vi "Fetch_chirp_waveform_optimized.vi"(0 "VISA resource name":refnum<visa-resource-name>, 11 "error in (no error)":errorcluster) -> (4 "VISA resource name out":refnum<visa-resource-name>, 6 "Waveform Data":waveform(dbl)(graph), 12 "overall meas time":u32, 15 "error out":errorcluster)   [LabVIEW 2011]
doc: "Returns the waveform that an oscilloscope acquires for a channel you specify. An acquisition that you initiate before calling this VI generates the waveform.\n\nYou first enable channels with the Configure Channel VI. Then you use the Initiate VI to start an acquisition on the enabled channels. An oscilloscope concurrently acquires waveforms for these channels. You must call the Fetch Waveform VI separately to obtain waveforms for each enabled channel. However, you also can call the Read Waveform VI instead of using the above low-level VIs.\n\n<B>Note:</B> Use the Fetch Waveform VI only with other low-level VIs, such as the Initiate VI, the Abort VI, and the Fetch Waveform Measurement VI. High-level VIs such as the Read Waveform VI automatically incorporate the functions of the Initiate VI and the Fetch Waveform VI. The Fetch Waveform VI does not check the status of an instrument."
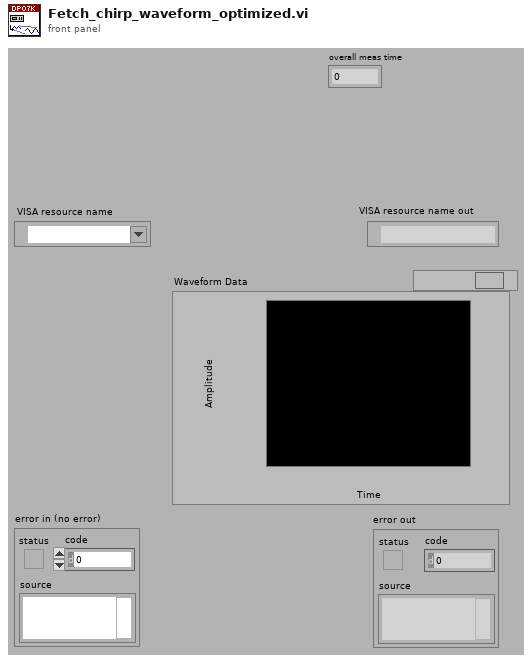
[diagram p1: front panel]
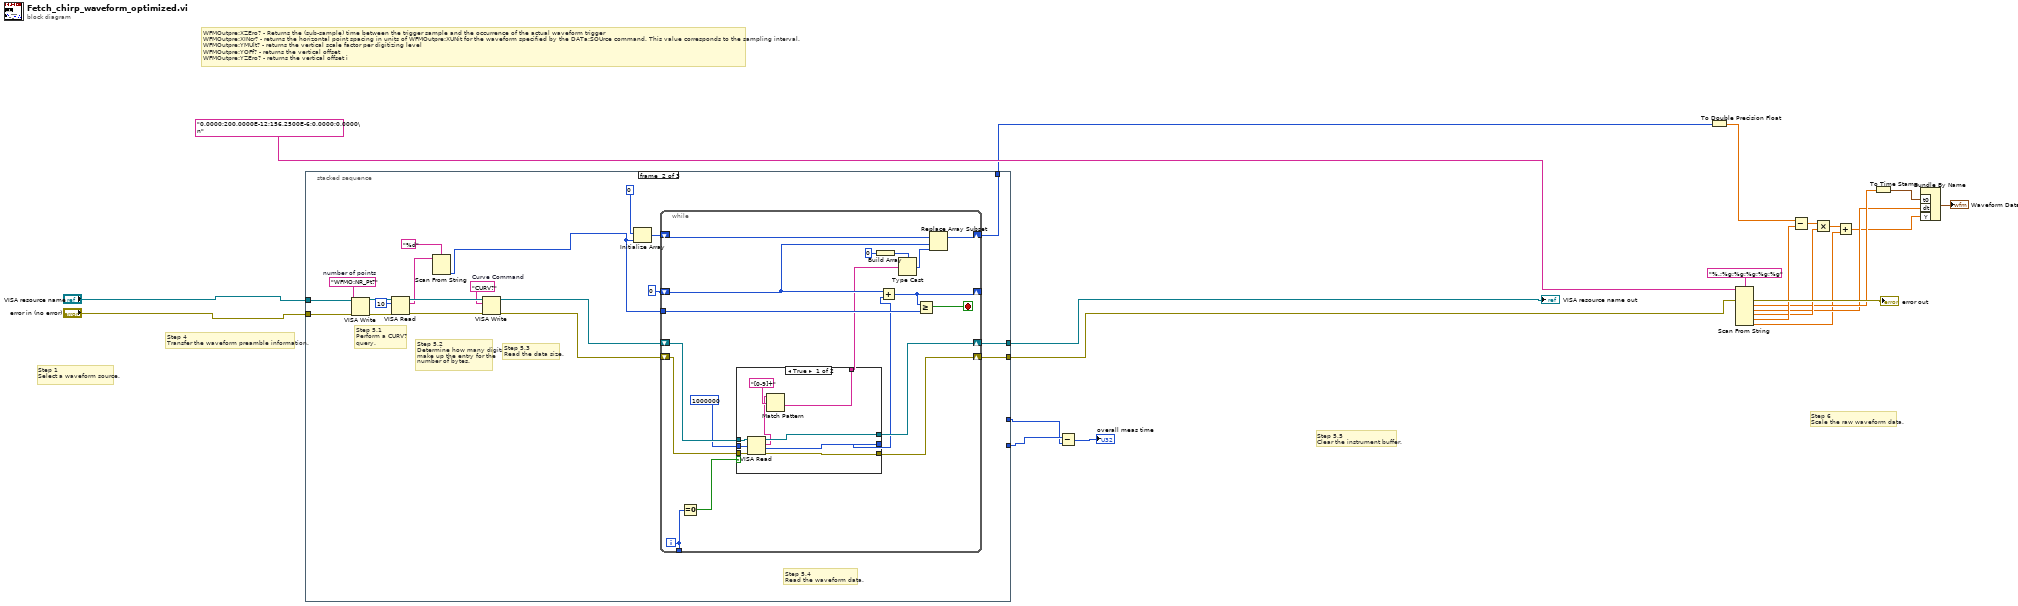
[diagram p0: block diagram]
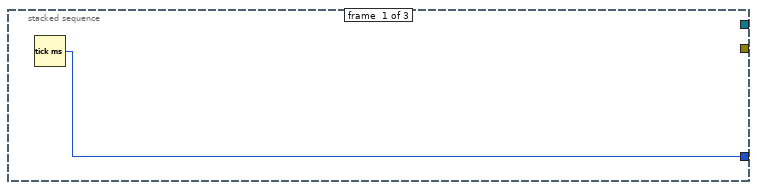
[diagram p2: hidden frame]
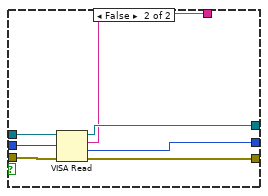
[diagram p3: hidden frame]
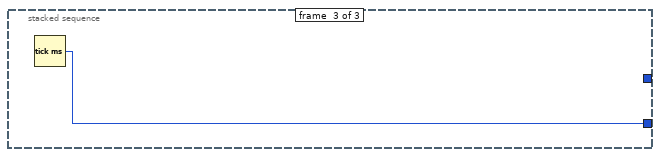
[diagram p4: hidden frame]
diagram:
  # "WFMOutpre:XZEro? - Returns the (sub-sample) time between the trigger sample and the occurrence of the actual waveform trigger\nWFMOutpre:XINcr? - returns the horizontal point spacing in units of WFMOutpre:XUNit for the waveform specified by the DATa:SOUrce command. This value corresponds to the sampling interval.\nWFMOutpre:YMUlt? - returns the vertical scale factor per digitizing level \nWFMOutpre:YOFf? - returns the vertical offset \nWFMOutpre:YZEro? - returns the vertical offset i"
  # "Step 1       \nSelect a waveform source."
  # "Step 6    \nScale the raw waveform data."
  # "Step 5.5    \nClear the instrument buffer."
  # "Step 4\nTransfer the waveform preamble information."
  n1 = stacked-sequence {
    tunnel: [_ w43 _] -> w21
    tunnel: [_ w42 _] -> w20
    tunnel: [_ w38 _] -> w18
    tunnel: "VISA resource name" -> [_ w37 _]
    tunnel: "error in (no error)" -> [_ w36 _]
    tunnel: [w23 _ _] -> w1
    tunnel: [_ _ w78] -> w2
    frame #0 {
      n2 = Tick Count (ms)() -> (millisecond timer value=w23:u32)
    }
    frame #1 {
      w24 = "CURV?"  # Curve Command
      w30 = "WFMO:NR_Pt?"  # number of points
      # "Step 5.4   \nRead the waveform data."
      # "Step 5.3      \nRead the data size."
      # "Step 5.2      \nDetermine how many digits\nmake up the entry for the \nnumber of bytes."
      # "Step 5.1      \nPerform a CURV?\nquery."
      n3 = VISA Write(VISA resource name=w37, write buffer=w30, error in (no error)=w36) -> (VISA resource name out=w31:refnum<visa-resource-name>, error out=w27:errorcluster)  [unwired: 1 out]
      n4 = VISA Read(VISA resource name=w31, byte count=u32 10, error in (no error)=w27) -> (VISA resource name out=w29:refnum<visa-resource-name>, read buffer=w25:string, error out=w28:errorcluster)  [unwired: 1 out]
      n5 = Scan From String(format string="%d", input string=w25) -> (output 1=w40:i32)  [unwired: 3 in, 3 out]
      n6 = VISA Write(VISA resource name=w29, write buffer=w24, error in (no error)=w28) -> (VISA resource name out=w41:refnum<visa-resource-name>, error out=w39:errorcluster)  [unwired: 1 out]
      n7 = Initialize Array(i8 0 ("element"), w40) -> (w34:i8[])
      n8 = while {
        shift-right: [w59] -> w42
        shift-left: w41 -> [w61]
        shift-right: [w58] -> w43
        shift-left: w39 -> [w48]
        shift-right: [w54] -> w38
        shift-left: w34 -> [w55]
        tunnel: w40 -> [w53]
        shift-right: [w50] -> _
        shift-left: 0 -> [w51]
        tunnel: [w45] -> _
        i -> [w45]
        stop <- w47 stop-if-true
        n9 = Equal To 0?(x=w45) -> (x = 0?=w44:bool)
        n10 = case shown="True" w44 {
          tunnel: w61 -> [w70 w77]
          tunnel: 1000000 ("Buffer Size") -> [w69 w76]
          tunnel: [w68 w75] -> w59
          tunnel: [w67 w74] -> w58
          tunnel: [w66 w73] -> w49
          tunnel: [w62 w72] -> w46
          tunnel: w48 -> [w65 w71]
          frame True {
            n11 = VISA Read(VISA resource name=w70, byte count=w69, error in (no error)=w65) -> (VISA resource name out=w68:refnum<visa-resource-name>, read buffer=w63:string, return count=w66:u32, error out=w67:errorcluster)
            n12 = Match Pattern(string=w63, regular expression="[0-9]+") -> (after substring=w62:string)  [unwired: 1 in, 3 out]
          }
          frame False {
            n13 = VISA Read(VISA resource name=w77, byte count=w76, error in (no error)=w71) -> (VISA resource name out=w75:refnum<visa-resource-name>, read buffer=w72:string, return count=w73:u32, error out=w74:errorcluster)
          }
        }
        n14 = Build Array(i8 0) -> (w57:i8[])
        n15 = Add(x=w51, y=w49) -> (x+y=w50:u32)
        n16 = Type Cast(type=w57, x=w46) -> (*(type *) &x=w52:i8[])
        n17 = Greater Or Equal?(x=w50, y=w53) -> (x >= y?=w47:bool)
        n18 = Replace Array Subset(array=w55, new element=w52, index=w51) -> (w54:i8[])
      }
    }
    frame #2 {
      n19 = Tick Count (ms)() -> (millisecond timer value=w78:u32)
    }
  }
  "VISA resource name out" <- w20
  n20 = Subtract(x=w2, y=w1) -> (x-y=→"overall meas time":u32)
  n21 = To Double Precision Float(number=w18) -> (double precision float=w19:dbl[])
  n22 = Scan From String(format string="%.;%g;%g;%g;%g;%g", input string="0.0000;200.0000E-12;156.2500E-6;0.0000;0.0000\n" ("read buffer"), error in=w21) -> (error out=→"error out":errorcluster, output 1=w11:dbl, output 2=w9:dbl, output 3=w13:dbl, output 4=w14:dbl, output 5=w7:dbl)  [unwired: 6 in, 2 out]
  n23 = Subtract(x=w19, y=w14) -> (x-y=w15:dbl[])
  n24 = Multiply(x=w15, y=w13) -> (x*y=w8:dbl[])
  n25 = Add(x=w8, y=w7) -> (x+y=w6:dbl[])
  n26 = To Time Stamp(1:w11) -> (0:w10:timestamp)
  n27 = Bundle By Name ("Build Waveform")("t0"=w10, "dt"=w9, "Y"=w6) -> (→"Waveform Data":waveform(dbl))  [unwired: 1 in]
